vi "Check FETs.vi"(8 "error in (no error)":errorcluster, 11 "MC VISA resource in":refnum<visa-resource-name>="ASRL1::INSTR") -> (0 "error out":errorcluster, 1 "FETs on?":bool=TRUE, 2 "Input E":bool=TRUE, 3 "VISA resource name out":refnum<visa-resource-name>, 5 "Emergency Stop":bool=TRUE)   [LabVIEW 2009]
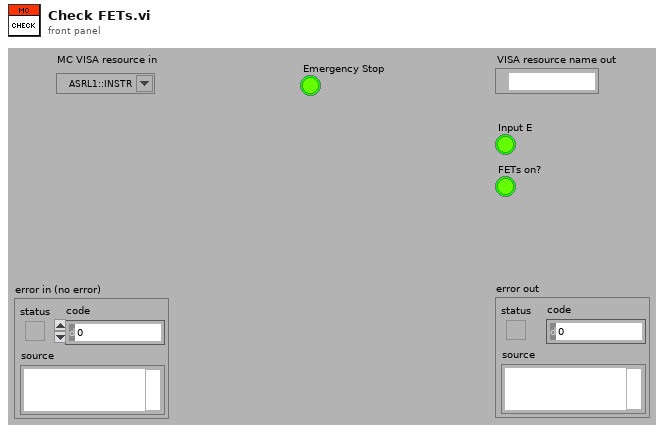
[diagram p1: front panel]
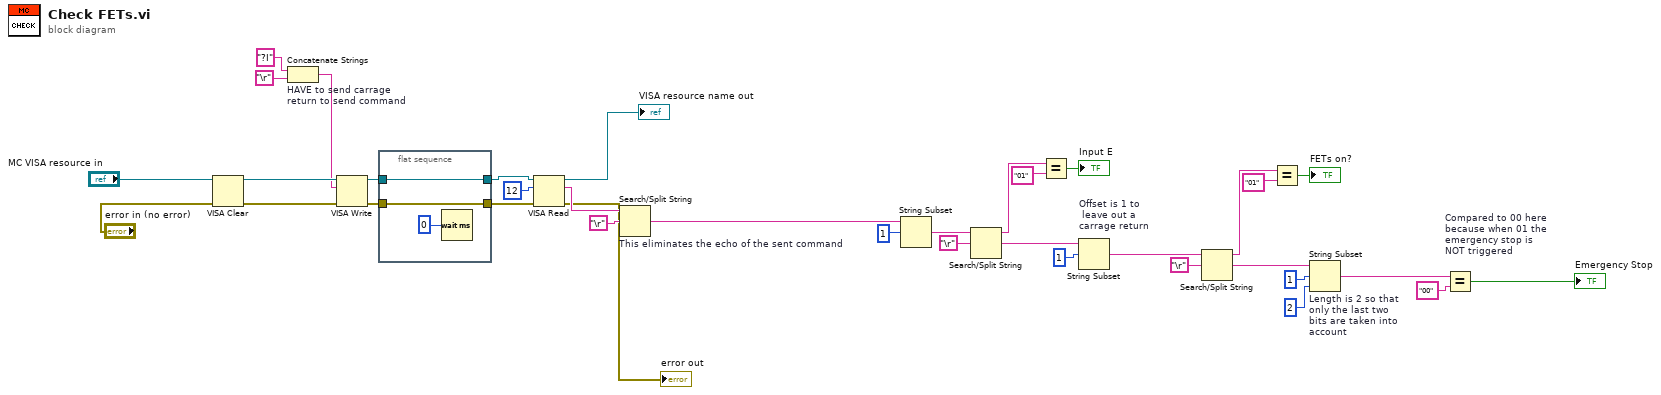
[diagram p0: block diagram]
diagram:
  n1 = VISA Clear(VISA resource name="MC VISA resource in", error in (no error)="error in (no error)") -> (VISA resource name out=w36:refnum<visa-resource-name>, error out=w35:errorcluster)
  n2 = Concatenate Strings "HAVE to send carrage\nreturn to send command"("?I" ("write buffer"), "\r") -> (w10:string)
  n3 = VISA Write(VISA resource name=w36, write buffer=w10, error in (no error)=w35) -> (VISA resource name out=w34:refnum<visa-resource-name>, error out=w32:errorcluster)  [unwired: 1 out]
  n4 = flat-sequence {
    tunnel: w34 -> [w39]
    tunnel: [w39] -> w33
    tunnel: w32 -> [w38]
    tunnel: [w38] -> w31
    frame #0 {
      n5 = Wait (ms)(milliseconds to wait=u32 0) -> ()  [unwired: 1 out]
    }
  }
  n6 = VISA Read(VISA resource name=w33, byte count=u32 12, error in (no error)=w31) -> (VISA resource name out=→"VISA resource name out":refnum<visa-resource-name>, read buffer=w9:string, error out=→"error out":errorcluster)  [unwired: 1 out]
  n7 = Search/Split String "This eliminates the echo of the sent command"(string=w9, search string/char (-)="\r") -> (match + rest of string=w7:string)  [unwired: 1 in, 2 out]
  n8 = String Subset(string=w7, offset (0)=1) -> (substring=w5:string)  [unwired: 1 in]
  n9 = Search/Split String(string=w5, search string/char (-)="\r") -> (substring before match=w29:string, match + rest of string=w26:string)  [unwired: 1 in, 1 out]
  n10 = Equal?(x=w29, y="01") -> (x = y?=→"Input E":bool)
  n11 = String Subset "Offset is 1 to\n leave out a \ncarrage return"(string=w26, offset (0)=1) -> (substring=w24:string)  [unwired: 1 in]
  n12 = Search/Split String(string=w24, search string/char (-)="\r") -> (substring before match=w22:string, match + rest of string=w19:string)  [unwired: 1 in, 1 out]
  n13 = Equal?(x=w22, y="01") -> (x = y?=→"FETs on?":bool)
  n14 = String Subset "Length is 2 so that\nonly the last two\nbits are taken into\naccount"(string=w19, offset (0)=1, length (rest)=2 ("length (rest)")) -> (substring=w16:string)
  n15 = Equal? "Compared to 00 here\nbecause when 01 the\nemergency stop is\nNOT triggered"(x=w16, y="00") -> (x = y?=→"Emergency Stop":bool)
